vi "Draw mObjects (SubVI).vi"(6 "Array":T1(array[cluster]), 9 "Math Values (Temporal)":sgl[](array[numeric]) format="%#.6g", 10 "Mimic mObjects":T2[](array[typedef]), 11 "picture in":picture) -> (3 "picture out":picture)   [LabVIEW 2014, in "SeqLoop.lvlib" / "Mimico Display.lvlib"]
uses:
  Mimico Display.lvlib
  TypeDefs/mObject.ctl
  <vilib>/regexp/Match Regular Expression.xnode
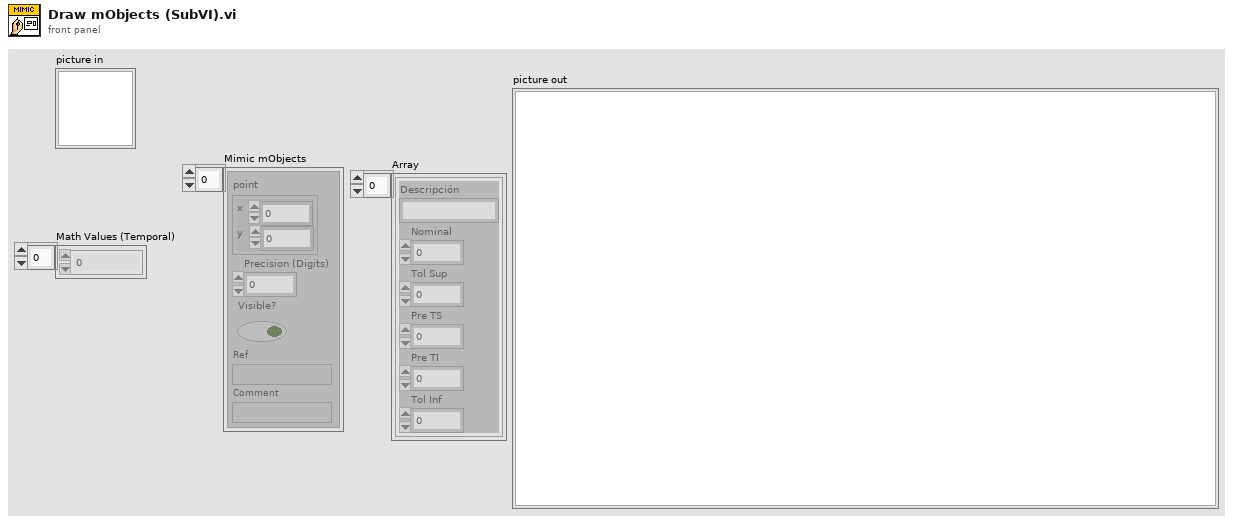
[diagram p1: front panel]
types:
  T1 = cluster{"Descripción":string, "Nominal":sgl, "Tol Sup":sgl, "Pre TS":sgl, "Pre TI":sgl, "Tol Inf":sgl}[]
  T2 = typedef "SeqLoop.lvlib/Mimico Display.lvlib/mObject.ctl" = cluster{"point":cluster{"x":i16, "y":i16}, "Precision (Digits)":i32, "Visible?":bool, "Ref":string, "Comment":string}
  T3 = cluster{"Descripción":string, "Nominal":i32, "Tol Sup":i32, "Pre TS":sgl, "Pre TI":i32, "Tol Inf":i32}
  T4 = cluster{"left":i16, "top":i16, "right":i16, "bottom":i16}
  T5 = cluster{"Width":i16, "Style":enum32{"Solid", "Dash", "Dot", "DashDot", "DashDotDot"}}
  T6 = enum16{"User-specified Font", "Application Font", "System Font", "Dialog Font"}
  T7 = cluster{"Font Name:":string, "Size":i16, "Strikeout?":bool, "Italic?":bool, "Underline?":bool, "Outline?":bool, "Shadow?":bool, "Bold?":bool}
  T8 = cluster{"horizontal":enum16{"left", "center", "right"}, "vertical":enum16{"top", "center", "bottom"}}
  T9 = cluster{"Descripción":string, "Nominal":sgl, "Tol Sup":sgl, "Pre TS":sgl, "Pre TI":sgl, "Tol Inf":sgl}
  T10 = typedef "imagedata.ctl" = cluster{"image type":i32, "image depth":i32, "image":u8[], "mask":u8[], "colors":u32[], "Rectangle":cluster{"left":i16, "top":i16, "right":i16, "bottom":i16}}
  T11 = cluster{"left":i16, "top":i16, i16, "bottom":i16}
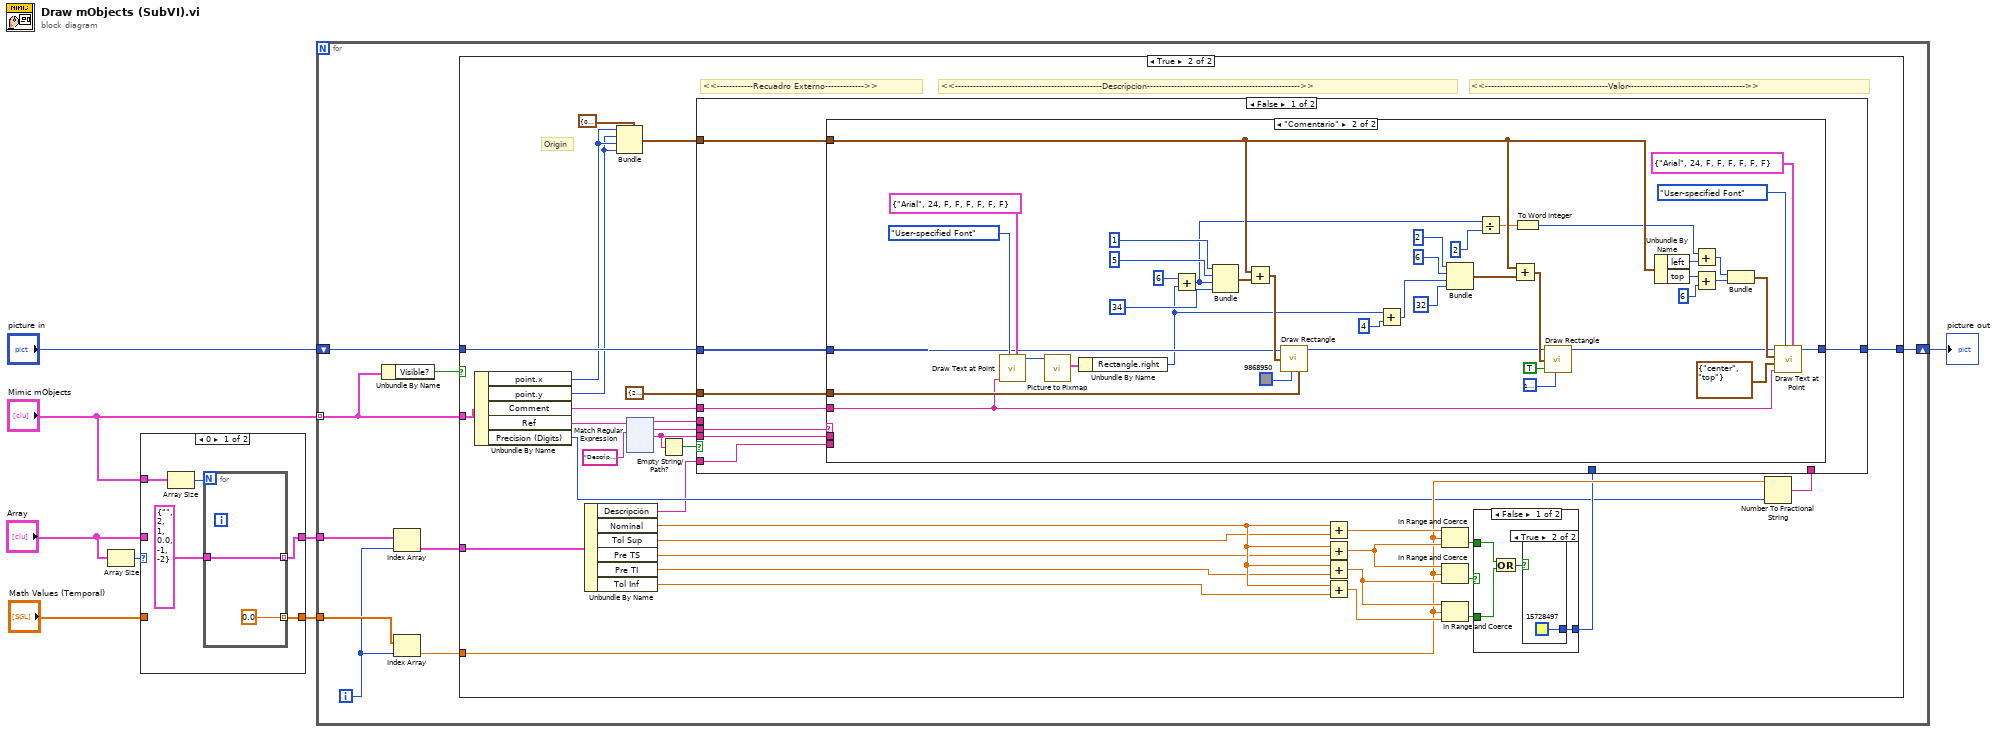
[diagram p0: block diagram]
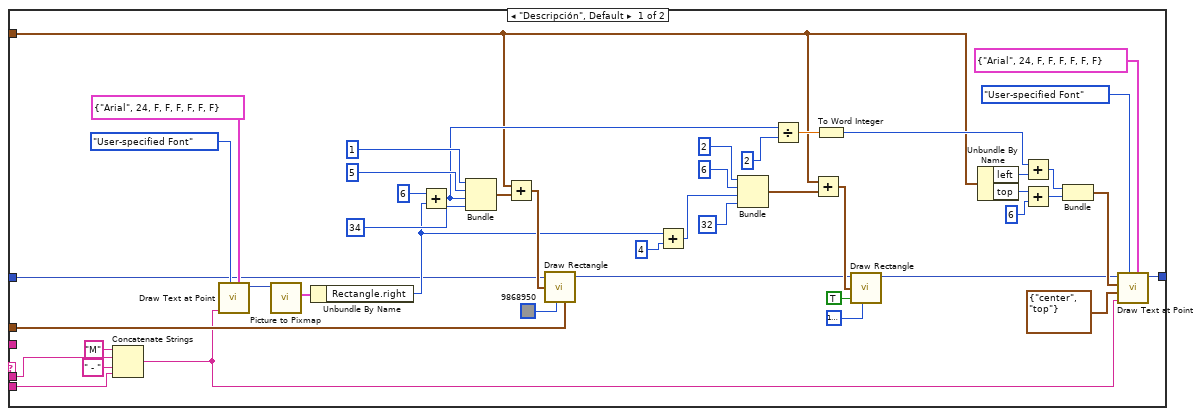
[diagram p4: hidden frame]
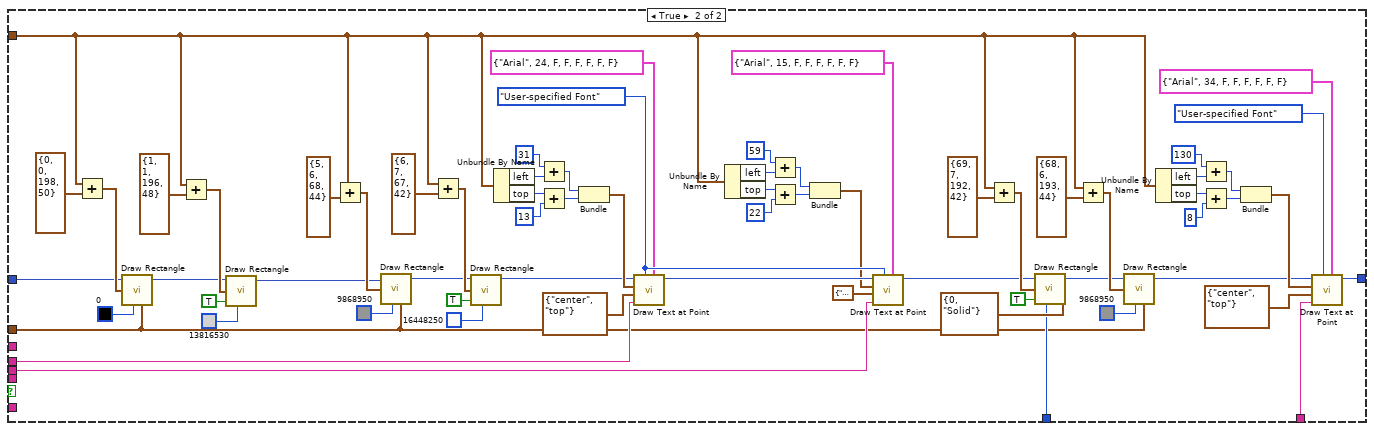
[diagram p5: hidden frame]
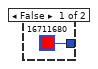
[diagram p6: hidden frame]
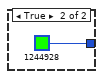
[diagram p7: hidden frame]
diagram:
  n1 = Array Size(array="Array") -> (size(s)=w2:i32)
  n2 = case shown="0" w2 {
    tunnel: "Array" -> [_ w17]
    tunnel: [w11 w17] -> w5
    tunnel: "Math Values (Temporal)" -> [_ w16]
    tunnel: [w9 w16] -> w3
    tunnel: "Mimic mObjects" -> [w13 _]
    frame 0 {
      n3 = Array Size(array=w13) -> (size(s)=w10:i32)
      n4 = for {
        N: w10 -> [_]
        tunnel: T3 {"Descripción"="", "Nominal"=2, "Tol Sup"=1, "Pre TS"=0.0, "Pre TI"=-1, "Tol Inf"=-2} ("output cluster") -> [w14]
        tunnel: [w14] -> w11 mode=indexing
        tunnel: [sgl 0.0] -> w9 mode=indexing
      }
    }
    frame 1, Default {
    }
  }
  n5 = for {
    tunnel: "Mimic mObjects" -> [w24] mode=indexing
    shift-right: [w25] -> w8
    shift-left: "picture in" -> [w26]
    tunnel: w5 -> [w19]
    tunnel: w3 -> [w22]
    i -> [w20]
    n6 = Unbundle By Name(w24) -> ("Visible?"=w23:bool)
    n7 = Index Array(array=w19, index=w20) -> (element=w18:T9)
    n8 = Index Array(array=w22, index=w20) -> (element=w21:sgl)
    n9 = case shown="True" w23 {
      tunnel: w24 -> [_ w60]
      tunnel: w26 -> [w27 w34]
      tunnel: [w27 w57] -> w25
      tunnel: w18 -> [_ w55]
      tunnel: w21 -> [_ w47]
      frame False {
      }
      frame True {
        # "<<-------------------------------------------------Descripcion--------------------------------------------------->>"
        # "<<-----------------------------------------Valor--------------------------------------->>"
        # "<<------------Recuadro Externo------------->>"
        # "Origin"
        n10 = Unbundle By Name(w60) -> ("point.x"=w32:i16, "point.y"=w30:i16, "Comment"=w31:string, "Ref"=w38:string, "Precision (Digits)"=w35:i32)
        n11 = Unbundle By Name(w55) -> ("Descripción"=w33:string, "Nominal"=w46:sgl, "Tol Sup"=w45:sgl, "Pre TS"=w44:sgl, "Pre TI"=w43:sgl, "Tol Inf"=w42:sgl)
        n12 = Bundle(cluster=T4 {"left"=0, "top"=0, "right"=0, "bottom"=0} ("rect"), "left"=w32, "top"=w30, "right"=w32, "bottom"=w30) -> (w39:T4)
        n13 = xnode "Match Regular Expression"("input string"=w38, "regular expression"="Descripción|Comentario|[0-9]+") -> ("before match"=w40:string, "whole match"=w37:string, "after match"=w28:string)  [unwired: 4 in, 2 out]
        n14 = Empty String/Path?(string/path=w28) -> (empty?=w36:bool)
        n15 = Add(x=w46, y=w45) -> (x+y=w48:sgl)
        n16 = Add(x=w46, y=w44) -> (x+y=w49:sgl)
        n17 = Add(x=w46, y=w43) -> (x+y=w50:sgl)
        n18 = Add(x=w46, y=w42) -> (x+y=w51:sgl)
        n19 = In Range and Coerce(upper limit=w48, x=w47, lower limit=w49) -> (In Range?=w53:bool)  [unwired: 1 out]
        n20 = In Range and Coerce(upper limit=w49, x=w47, lower limit=w50) -> (In Range?=w54:bool)  [unwired: 1 out]
        n21 = In Range and Coerce(upper limit=w50, x=w47, lower limit=w51) -> (In Range?=w52:bool)  [unwired: 1 out]
        n22 = case shown="False" w54 {
          tunnel: w53 -> [w337 _]
          tunnel: w52 -> [w336 _]
          tunnel: [w335 u32 1244928] -> w41
          frame False {
            n23 = Or(x=w337, y=w336) -> (x .or. y?=w338:bool)
            n24 = case shown="True" w338 {
              tunnel: [u32 16711680 u32 15728497] -> w335
              frame False {
              }
              frame True {
              }
            }
          }
          frame True {
          }
        }
        n25 = Number To Fractional String(number=w47, precision (6)=w35) -> (F-format string=w56:string)  [unwired: 2 in]
        n26 = case shown="False" w36 {
          tunnel: T5 {"Width"=2, "Style"=enum."Solid"} ("pen") -> [w67 w155]
          tunnel: [w66 w209] -> w57
          tunnel: w56 -> [_ w201]
          tunnel: w34 -> [w65 w157]
          tunnel: w41 -> [_ w199]
          tunnel: w40 -> [_ w182]
          tunnel: w39 -> [w68 w156]
          tunnel: w37 -> [w62 w176]
          tunnel: w31 -> [w61 _]
          tunnel: w33 -> [w64 _]
          tunnel: w28 -> [w63 _]
          frame False {
            n27 = case shown="\"Comentario\"" w62 {
              tunnel: w68 -> [w75 w138]
              tunnel: w67 -> [w77 w137]
              tunnel: [w74 w136] -> w66
              tunnel: w65 -> [w76 w122]
              tunnel: w64 -> [w70 _]
              tunnel: w63 -> [w73 _]
              tunnel: w61 -> [_ w114]
              frame "Descripción", Default {
                n28 = Concatenate Strings("M" ("string"), w73, " - " ("string"), w70) -> (w71:string)
                n29 = call <vilib>:"Draw Text at Point.vi"("[user-specified font]"=T7 {"Font Name:"="Arial", "Size"=24, "Strikeout?"=FALSE, "Italic?"=FALSE, "Underline?"=FALSE, "Outline?"=FALSE, "Shadow?"=FALSE, "Bold?"=FALSE}, "desired font(Application)"=T6."User-specified Font", "text"=w71) -> ("new picture"=w84:picture)  [unwired: 7 in, 1 out]
                n30 = call <vilib>:"Picture to Pixmap.vi"("picture"=w84) -> ("image data"=w83:T10)  [unwired: 9 in, 1 out]
                n31 = Unbundle By Name(w83) -> ("Rectangle.right"=w79:i16)
                n32 = Add(x=i16 6, y=w79) -> (x+y=w78:i16)
                n33 = Bundle("left"=i16 1, "top"=i16 5, w78, "bottom"=i16 34) -> (w95:T11)  [unwired: 1 in]
                n34 = Add(x=w75, y=w95) -> (x+y=w106:T11)
                n35 = call <vilib>:"Draw Rectangle.vi"("picture"=w76, "rect"=w106, "color(black)"=u32 9868950, "pen"=w77) -> ("new picture"=w102:picture)  [unwired: 5 in]
                n36 = Add(x=w79, y=i16 4) -> (x+y=w80:i16)
                n37 = Bundle("left"=i16 2, "top"=i16 6, w80, "bottom"=i16 32) -> (w91:T11)  [unwired: 1 in]
                n38 = Divide(x=w78, y=i16 2 ("left")) -> (x/y=w88:dbl)
                n39 = Add(x=w75, y=w91) -> (x+y=w104:T11)
                n40 = To Word Integer(number=w88) -> (16bit integer=w87:i16)
                n41 = call <vilib>:"Draw Rectangle.vi"("picture"=w102, "rect"=w104, "fill?(F)"=TRUE, "color(black)"=u32 16777216) -> ("new picture"=w107:picture)  [unwired: 5 in]
                n42 = Unbundle By Name(w75) -> ("left"=w112:i16, "top"=w109:i16)
                n43 = Add(x=w87, y=w112) -> (x+y=w111:i16)
                n44 = Add(x=w109, y=i16 6 ("x")) -> (x+y=w108:i16)
                n45 = Bundle(w111, w108) -> (w113:cluster{i16, i16})  [unwired: 1 in]
                n46 = call <vilib>:"Draw Text at Point.vi"("[user-specified font]"=T7 {"Font Name:"="Arial", "Size"=24, "Strikeout?"=FALSE, "Italic?"=FALSE, "Underline?"=FALSE, "Outline?"=FALSE, "Shadow?"=FALSE, "Bold?"=FALSE}, "desired font(Application)"=T6."User-specified Font", "text"=w71, "alignment(left, top)"=T8 {"horizontal"=enum."center", "vertical"=enum."top"}, "origin"=w113, "picture"=w107) -> ("new picture"=w74:picture)  [unwired: 4 in, 1 out]
              }
              frame "Comentario" {
                n47 = call <vilib>:"Draw Text at Point.vi"("[user-specified font]"=T7 {"Font Name:"="Arial", "Size"=24, "Strikeout?"=FALSE, "Italic?"=FALSE, "Underline?"=FALSE, "Outline?"=FALSE, "Shadow?"=FALSE, "Bold?"=FALSE}, "desired font(Application)"=T6."User-specified Font", "text"=w114) -> ("new picture"=w121:picture)  [unwired: 7 in, 1 out]
                n48 = call <vilib>:"Picture to Pixmap.vi"("picture"=w121) -> ("image data"=w120:T10)  [unwired: 9 in, 1 out]
                n49 = Unbundle By Name(w120) -> ("Rectangle.right"=w116:i16)
                n50 = Add(x=i16 6, y=w116) -> (x+y=w115:i16)
                n51 = Bundle("left"=i16 1, "top"=i16 5, w115, "bottom"=i16 34) -> (w133:T11)  [unwired: 1 in]
                n52 = Add(x=w138, y=w133) -> (x+y=w147:T11)
                n53 = call <vilib>:"Draw Rectangle.vi"("picture"=w122, "rect"=w147, "color(black)"=u32 9868950, "pen"=w137) -> ("new picture"=w143:picture)  [unwired: 5 in]
                n54 = Add(x=w116, y=i16 4) -> (x+y=w117:i16)
                n55 = Bundle("left"=i16 2, "top"=i16 6, w117, "bottom"=i16 32) -> (w129:T11)  [unwired: 1 in]
                n56 = Divide(x=w115, y=i16 2 ("left")) -> (x/y=w126:dbl)
                n57 = Add(x=w138, y=w129) -> (x+y=w145:T11)
                n58 = To Word Integer(number=w126) -> (16bit integer=w125:i16)
                n59 = call <vilib>:"Draw Rectangle.vi"("picture"=w143, "rect"=w145, "fill?(F)"=TRUE, "color(black)"=u32 16777216) -> ("new picture"=w148:picture)  [unwired: 5 in]
                n60 = Unbundle By Name(w138) -> ("left"=w153:i16, "top"=w150:i16)
                n61 = Add(x=w125, y=w153) -> (x+y=w152:i16)
                n62 = Add(x=w150, y=i16 6 ("x")) -> (x+y=w149:i16)
                n63 = Bundle(w152, w149) -> (w154:cluster{i16, i16})  [unwired: 1 in]
                n64 = call <vilib>:"Draw Text at Point.vi"("[user-specified font]"=T7 {"Font Name:"="Arial", "Size"=24, "Strikeout?"=FALSE, "Italic?"=FALSE, "Underline?"=FALSE, "Outline?"=FALSE, "Shadow?"=FALSE, "Bold?"=FALSE}, "desired font(Application)"=T6."User-specified Font", "text"=w114, "alignment(left, top)"=T8 {"horizontal"=enum."center", "vertical"=enum."top"}, "origin"=w154, "picture"=w148) -> ("new picture"=w136:picture)  [unwired: 4 in, 1 out]
              }
            }
          }
          frame True {
            w179 = T6."User-specified Font" ("desired font(Application)")
            n65 = Add(x=w156, y=T4 {"left"=0, "top"=0, "right"=198, "bottom"=50} ("rect")) -> (x+y=w165:T4)
            n66 = call <vilib>:"Draw Rectangle.vi"("picture"=w157, "rect"=w165, "color(black)"=u32 0, "pen"=w155) -> ("new picture"=w161:picture)  [unwired: 5 in]
            n67 = Add(x=w156, y=T4 {"left"=1, "top"=1, "right"=196, "bottom"=48} ("rect")) -> (x+y=w163:T4)
            n68 = call <vilib>:"Draw Rectangle.vi"("picture"=w161, "rect"=w163, "fill?(F)"=TRUE, "color(black)"=u32 13816530) -> ("new picture"=w158:picture)  [unwired: 5 in]
            n69 = Add(x=w156, y=T4 {"left"=5, "top"=6, "right"=68, "bottom"=44} ("rect")) -> (x+y=w189:T4)
            n70 = call <vilib>:"Draw Rectangle.vi"("picture"=w158, "rect"=w189, "color(black)"=u32 9868950, "pen"=w155) -> ("new picture"=w184:picture)  [unwired: 5 in]
            n71 = Add(x=w156, y=T4 {"left"=6, "top"=7, "right"=67, "bottom"=42} ("rect")) -> (x+y=w187:T4)
            n72 = call <vilib>:"Draw Rectangle.vi"("picture"=w184, "rect"=w187, "fill?(F)"=TRUE, "color(black)"=u32 16448250) -> ("new picture"=w191:picture)  [unwired: 5 in]
            n73 = Unbundle By Name(w156) -> ("left"=w197:i16, "top"=w193:i16)
            n74 = Add(x=i16 31, y=w197) -> (x+y=w196:i16)
            n75 = Add(x=w193, y=i16 13 ("x")) -> (x+y=w192:i16)
            n76 = Bundle(w196, w192) -> (w198:cluster{i16, i16})  [unwired: 1 in]
            n77 = call <vilib>:"Draw Text at Point.vi"("[user-specified font]"=T7 {"Font Name:"="Arial", "Size"=24, "Strikeout?"=FALSE, "Italic?"=FALSE, "Underline?"=FALSE, "Outline?"=FALSE, "Shadow?"=FALSE, "Bold?"=FALSE}, "desired font(Application)"=w179, "text"=w182, "alignment(left, top)"=T8 {"horizontal"=enum."center", "vertical"=enum."top"}, "origin"=w198, "picture"=w191) -> ("new picture"=w181:picture)  [unwired: 4 in, 1 out]
            n78 = Unbundle By Name(w156) -> ("left"=w170:i16, "top"=w174:i16)
            n79 = Add(x=i16 59, y=w170) -> (x+y=w171:i16)
            n80 = Add(x=w174, y=i16 22 ("x")) -> (x+y=w175:i16)
            n81 = Bundle(w171, w175) -> (w169:cluster{i16, i16})  [unwired: 1 in]
            n82 = call <vilib>:"Draw Text at Point.vi"("[user-specified font]"=T7 {"Font Name:"="Arial", "Size"=15, "Strikeout?"=FALSE, "Italic?"=FALSE, "Underline?"=FALSE, "Outline?"=FALSE, "Shadow?"=FALSE, "Bold?"=FALSE}, "desired font(Application)"=w179, "text"=w176, "alignment(left, top)"=T8 {"horizontal"=enum."center", "vertical"=enum."top"}, "origin"=w169, "picture"=w181) -> ("new picture"=w180:picture)  [unwired: 4 in, 1 out]
            n83 = Add(x=w156, y=T4 {"left"=69, "top"=7, "right"=192, "bottom"=42} ("rect")) -> (x+y=w207:T4)
            n84 = call <vilib>:"Draw Rectangle.vi"("picture"=w180, "rect"=w207, "fill?(F)"=TRUE, "color(black)"=w199, "pen"=T5 {"Width"=0, "Style"=enum."Solid"}) -> ("new picture"=w205:picture)  [unwired: 4 in]
            n85 = Add(x=w156, y=T4 {"left"=68, "top"=6, "right"=193, "bottom"=44} ("rect")) -> (x+y=w214:T4)
            n86 = call <vilib>:"Draw Rectangle.vi"("picture"=w205, "rect"=w214, "color(black)"=u32 9868950, "pen"=w155) -> ("new picture"=w210:picture)  [unwired: 5 in]
            n87 = Unbundle By Name(w156) -> ("left"=w215:i16, "top"=w219:i16)
            n88 = Add(x=i16 130, y=w215) -> (x+y=w216:i16)
            n89 = Add(x=w219, y=i16 8 ("x")) -> (x+y=w220:i16)
            n90 = Bundle(w216, w220) -> (w213:cluster{i16, i16})  [unwired: 1 in]
            n91 = call <vilib>:"Draw Text at Point.vi"("[user-specified font]"=T7 {"Font Name:"="Arial", "Size"=34, "Strikeout?"=FALSE, "Italic?"=FALSE, "Underline?"=FALSE, "Outline?"=FALSE, "Shadow?"=FALSE, "Bold?"=FALSE}, "desired font(Application)"=T6."User-specified Font", "text"=w201, "alignment(left, top)"=T8 {"horizontal"=enum."center", "vertical"=enum."top"}, "origin"=w213, "picture"=w210) -> ("new picture"=w209:picture)  [unwired: 4 in, 1 out]
          }
        }
      }
    }
  }
  "picture out" <- w8
